vi "MIDI command to playback state.vi"(10 "Track Controls":T1={"Track 0"={"Effects Settings"={"Delay"=4.86522497566e-313, "Delay 2"=4.86522497566e-313}, "Volume Settings"={"Mute"=FALSE, "Solo"=FALSE, "Record"=FALSE, "Pan"=4.86522497566e-313, "Volume"=4.86522497566e-313}}, "Track 1"={"Effects Settings"={"Delay"=0.0, "Delay 2"=0.0}, "Volume Settings"={"Mute"=FALSE, "Solo"=FALSE, "Record"=FALSE, "Pan"=0.0, "Volume"=0.0}}, "Track 2"={"Effects Settings"={"Delay"=0.0, "Delay 2"=0.0}, "Volume Settings"={"Mute"=FALSE, "Solo"=FALSE, "Record"=FALSE, "Pan"=0.0, "Volume"=0.0}}, "Track 3"={"Effects Settings"={"Delay"=0.0, "Delay 2"=0.0}, "Volume Settings"={"Mute"=FALSE, "Solo"=FALSE, "Record"=FALSE, "Pan"=0.0, "Volume"=0.0}}} {"Track 3"."Volume Settings"."Volume" scale=1.0..10.0; "Track 3"."Volume Settings"."Pan" scale=0.0..1.0; "Track 3"."Effects Settings"."Delay 2" scale=0.0..10.0; "Track 3"."Effects Settings"."Delay" scale=0.0..1.0; "Track 2"."Volume Settings"."Volume" scale=1.0..10.0; "Track 2"."Volume Settings"."Pan" scale=0.0..1.0; "Track 2"."Effects Settings"."Delay 2" scale=0.0..10.0; "Track 2"."Effects Settings"."Delay" scale=0.0..1.0; "Track 1"."Volume Settings"."Volume" scale=1.0..10.0; "Track 1"."Volume Settings"."Pan" scale=0.0..1.0; "Track 1"."Effects Settings"."Delay 2" scale=0.0..10.0; "Track 1"."Effects Settings"."Delay" scale=0.0..1.0; "Track 0"."Volume Settings"."Volume" scale=1.0..10.0; "Track 0"."Volume Settings"."Pan" scale=0.0..1.0; "Track 0"."Effects Settings"."Delay 2" scale=0.0..10.0; "Track 0"."Effects Settings"."Delay" scale=0.0..1.0}, 11 "Midi Command":T6) -> (2 "Track Controls":T1={"Track 0"={"Effects Settings"={"Delay"=4.86522497566e-313, "Delay 2"=4.86522497566e-313}, "Volume Settings"={"Mute"=FALSE, "Solo"=FALSE, "Record"=FALSE, "Pan"=4.86522497566e-313, "Volume"=4.86522497566e-313}}, "Track 1"={"Effects Settings"={"Delay"=0.0, "Delay 2"=0.0}, "Volume Settings"={"Mute"=FALSE, "Solo"=FALSE, "Record"=FALSE, "Pan"=0.0, "Volume"=0.0}}, "Track 2"={"Effects Settings"={"Delay"=0.0, "Delay 2"=0.0}, "Volume Settings"={"Mute"=FALSE, "Solo"=FALSE, "Record"=FALSE, "Pan"=0.0, "Volume"=0.0}}, "Track 3"={"Effects Settings"={"Delay"=0.0, "Delay 2"=0.0}, "Volume Settings"={"Mute"=FALSE, "Solo"=FALSE, "Record"=FALSE, "Pan"=0.0, "Volume"=0.0}}} {"Track 3"."Volume Settings"."Volume" scale=1.0..10.0; "Track 3"."Volume Settings"."Pan" scale=0.0..1.0; "Track 3"."Effects Settings"."Delay 2" scale=0.0..10.0; "Track 3"."Effects Settings"."Delay" scale=0.0..1.0; "Track 2"."Volume Settings"."Volume" scale=1.0..10.0; "Track 2"."Volume Settings"."Pan" scale=0.0..1.0; "Track 2"."Effects Settings"."Delay 2" scale=0.0..10.0; "Track 2"."Effects Settings"."Delay" scale=0.0..1.0; "Track 1"."Volume Settings"."Volume" scale=1.0..10.0; "Track 1"."Volume Settings"."Pan" scale=0.0..1.0; "Track 1"."Effects Settings"."Delay 2" scale=0.0..10.0; "Track 1"."Effects Settings"."Delay" scale=0.0..1.0; "Track 0"."Volume Settings"."Volume" scale=1.0..10.0; "Track 0"."Volume Settings"."Pan" scale=0.0..1.0; "Track 0"."Effects Settings"."Delay 2" scale=0.0..10.0; "Track 0"."Effects Settings"."Delay" scale=0.0..1.0}, 3 "Next State":T5)   [LabVIEW 2014]
uses:
  MIDI/Controls/MidiCommand.ctl
  Controls/playback state.ctl
  Controls/Track Controls.ctl
  Controls/Track Settings.ctl
  Controls/Track Effects Settings.ctl
  Controls/Track Volume Settings.ctl
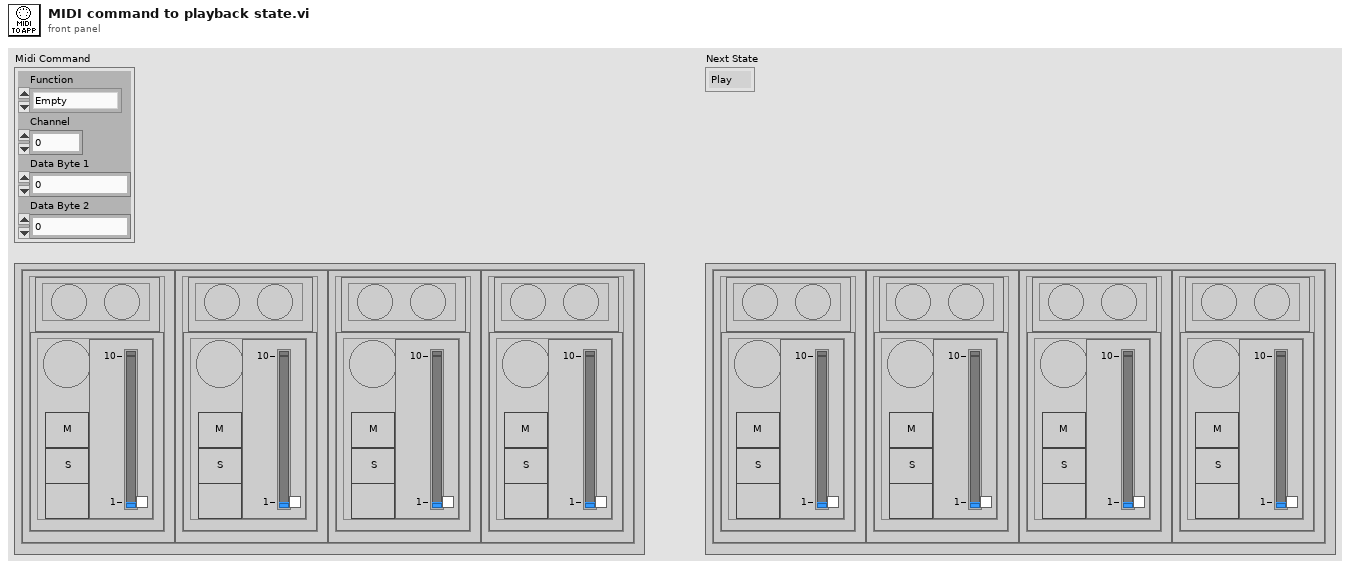
[diagram p1: front panel]
types:
  T1 = typedef "Track Controls.ctl" = cluster{"Track 0":T2, "Track 1":T2, "Track 2":T2, "Track 3":T2}
  T2 = typedef "Track Settings.ctl" = cluster{"Effects Settings":T3, "Volume Settings":T4}
  T3 = typedef "Track Effects Settings.ctl" = cluster{"Delay":dbl, "Delay 2":dbl}
  T4 = typedef "Track Volume Settings.ctl" = cluster{"Mute":bool, "Solo":bool, "Record":bool, "Pan":dbl, "Volume":dbl}
  T5 = typedef "playback state.ctl" = enum16{"Play", "Record", "Stop", "Pause", "Rewind"}
  T6 = typedef "MidiCommand.ctl" = cluster{"Function":enum16{"Empty", "Note Off", "Note On", "Polyphonic Aftertouch", "Control/Mode Change", "Program Change", "Channel Aftertouch", "Pitch Bend Change", "System"}, "Channel":u8, "Data Byte 1":u8, "Data Byte 2":u8}
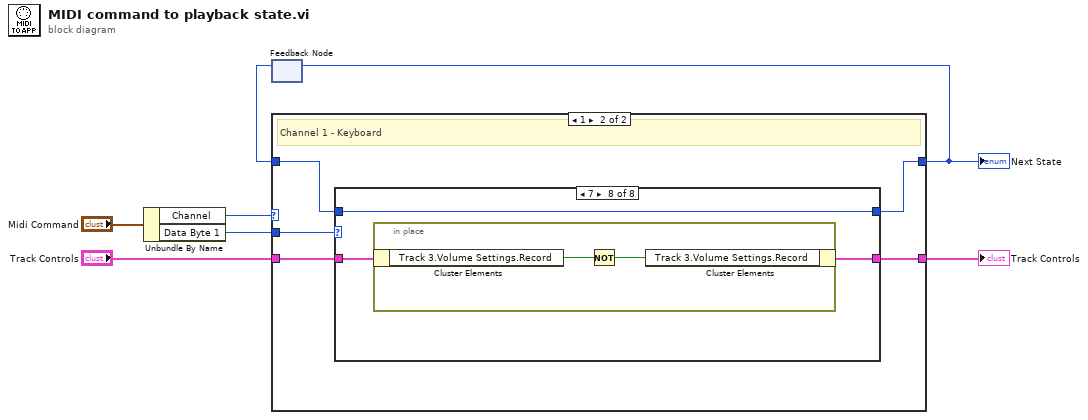
[diagram p0: block diagram]
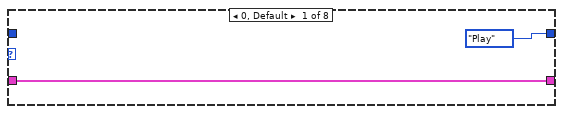
[diagram p3: hidden frame]
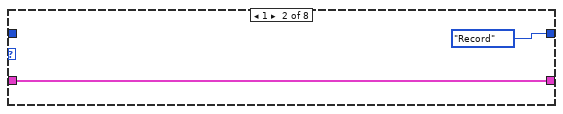
[diagram p4: hidden frame]
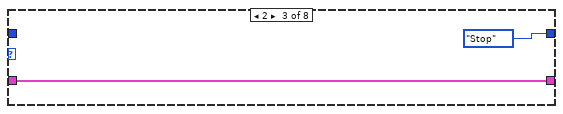
[diagram p5: hidden frame]
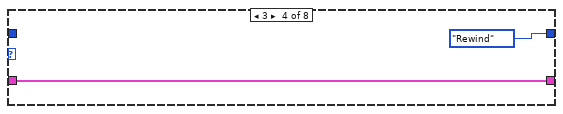
[diagram p6: hidden frame]
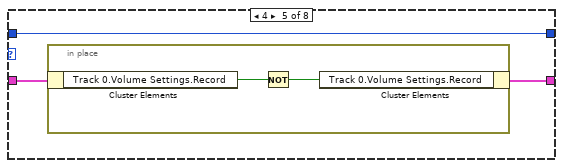
[diagram p7: hidden frame]
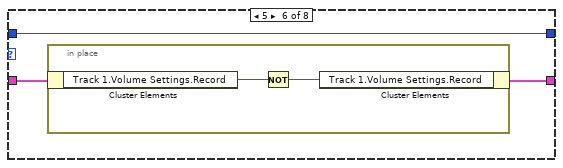
[diagram p8: hidden frame]
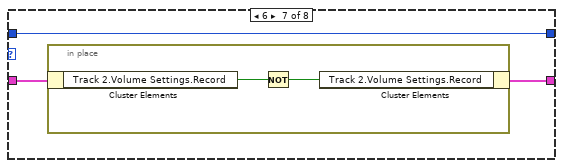
[diagram p9: hidden frame]
diagram:
  n1 = Unbundle By Name("Midi Command") -> ("Channel"=w6:u8, "Data Byte 1"=w5:u8)
  n2 = feedback #1() -> (w3:T5)  [unwired: 1 in]
  n3 = case shown="1" w6 {
    tunnel: w5 -> [_ w14]
    tunnel: [w9 w13] -> w4
    tunnel: w3 -> [w9 w12]
    tunnel: "Track Controls" -> [w8 w11]
    tunnel: [w8 w10] -> w1
    frame 0, Default {
    }
    frame 1 {
      # "Channel 1 - Keyboard"
      n4 = case shown="7" w14 {
        tunnel: [playback_state."Play" ("Next State") playback_state."Record" ("Next State") playback_state."Stop" ("Next State") playback_state."Rewind" ("Next State") w25 w30 w35 w40] -> w13
        tunnel: w12 -> [_ _ _ _ w25 w30 w35 w40]
        tunnel: w11 -> [w15 w17 w19 w21 w24 w29 w34 w39]
        tunnel: [w15 w17 w19 w21 w23 w28 w33 w38] -> w10
        frame 0, Default {
        }
        frame 1 {
        }
        frame 2 {
        }
        frame 3 {
        }
        frame 4 {
          n5 = in-place {
            n6 = in-place-cluster #2(w24) -> ("Track 0.Volume Settings.Record"=w27:bool)
            n7 = Not(x=w27) -> (.not. x?=w26:bool)
            n8 = in-place-cluster #2("Track 0.Volume Settings.Record"=w26) -> (w23:T1)
          }
        }
        frame 5 {
          n9 = in-place {
            n10 = in-place-cluster #3(w29) -> ("Track 1.Volume Settings.Record"=w32:bool)
            n11 = Not(x=w32) -> (.not. x?=w31:bool)
            n12 = in-place-cluster #3("Track 1.Volume Settings.Record"=w31) -> (w28:T1)
          }
        }
        frame 6 {
          n13 = in-place {
            n14 = in-place-cluster #4(w34) -> ("Track 2.Volume Settings.Record"=w37:bool)
            n15 = Not(x=w37) -> (.not. x?=w36:bool)
            n16 = in-place-cluster #4("Track 2.Volume Settings.Record"=w36) -> (w33:T1)
          }
        }
        frame 7 {
          n17 = in-place {
            n18 = in-place-cluster #5(w39) -> ("Track 3.Volume Settings.Record"=w42:bool)
            n19 = Not(x=w42) -> (.not. x?=w41:bool)
            n20 = in-place-cluster #5("Track 3.Volume Settings.Record"=w41) -> (w38:T1)
          }
        }
      }
    }
  }
  "Next State" <- w4
  "Track Controls" <- w1
  n21 = feedback-in #1(w4) -> ()
